vi "ReadXCANVersion.vi"() -> (1 "InstallTime":string, 2 "Version":string)   [LabVIEW 2015]
uses:
  <vilib>/registry/registry.llb/Registry RtKey.ctl
  <vilib>/registry/registry.llb/Registry SAM.ctl
  <vilib>/registry/registry.llb/Registry View.ctl
  <vilib>/registry/registry.llb/Read Registry Value Simple STR.vi
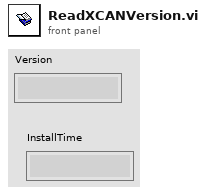
[diagram p1: front panel]
types:
  T1 = typedef "Registry View.ctl" = u16
  T2 = typedef "Registry SAM.ctl" = enum32{"KEY_QUERY_VALUE", "KEY_SET_VALUE", "KEY_CREATE_SUB_KEY", "KEY_ENUMERATE_SUB_KEYS", "KEY_NOTIFY", "KEY_CREATE_LINK", "KEY_READ", "KEY_WRITE", "KEY_ALL_ACCESS", "KEY_READ | KEY_WRITE"}
  T3 = typedef "Registry RtKey.ctl" = enum32{"HKEY_CLASSES_ROOT", "HKEY_CURRENT_USER", "HKEY_LOCAL_MACHINE", "HKEY_USERS", "HKEY_PERFORMANCE_DATA", "HKEY_CURRENT_CONFIG", "HKEY_DYN_DATA"}
  T4 = typedef "Registry refnum.ctl" = refnum<k1>
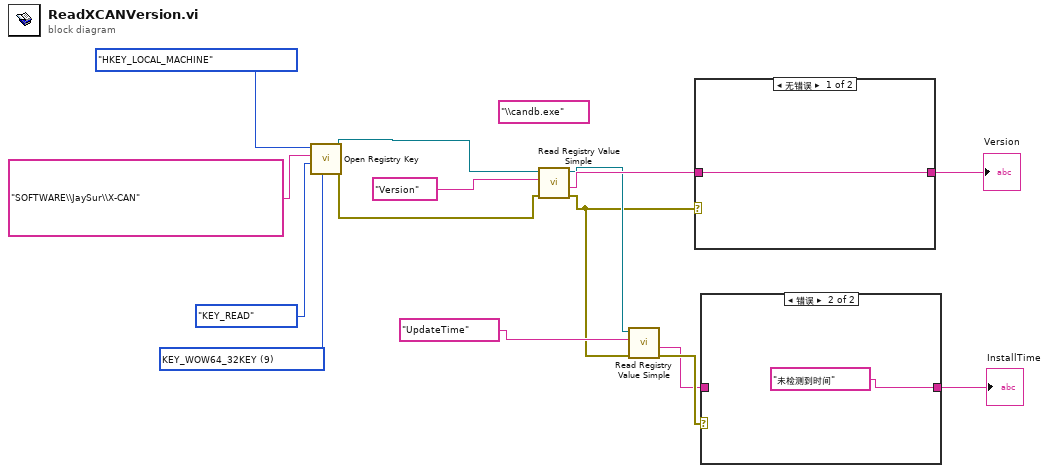
[diagram p0: block diagram]
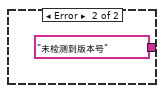
[diagram p3: hidden frame]
diagram:
  (unwired) "\\candb.exe" ("字符串")
  w12 = T1 9 items=["Default"=0, "KEY_WOW64_64KEY"=8, "KEY_WOW64_32KEY"=9] ("registry view")
  n1 = call <vilib>:"Open Registry Key.vi"("registry view"=w12, "security access mask (KEY_READ | KEY_WRITE)"=Registry_SAM."KEY_READ", "subkey"="SOFTWARE\\JaySur\\X-CAN", "root key (HKEY_LOCAL_MACHINE)"=Registry_RtKey."HKEY_LOCAL_MACHINE") -> ("error out"=w9:errorcluster, "refnum out"=w11:T4)  [unwired: 6 in]
  n2 = call-poly <vilib>:"Read Registry Value Simple.vi"("error in (no error)"=w9, "value"="Version", "refnum"=w11) -> ("error out"=w4:errorcluster, "String/Binary data"=w8:string, "refnum out"=w6:T4)  [unwired: 3 in, 1 out]
  n3 = call-poly <vilib>:"Read Registry Value Simple.vi"("error in (no error)"=w4, "value"="UpdateTime", "refnum"=w6) -> ("error out"=w3:errorcluster, "String/Binary data"=w2:string)  [unwired: 3 in, 2 out]
  n4 = case shown="无错误" w4 {
    tunnel: w8 -> [w16 _]
    tunnel: [w16 "未检测到版本号" ("String/Binary data")] -> w7
    frame No Error {
    }
    frame Error {
    }
  }
  "Version" <- w7
  n5 = case shown="错误" w3 {
    tunnel: w2 -> [w18 _]
    tunnel: [w18 "未检测到时间" ("String/Binary data")] -> w1
    frame No Error {
    }
    frame Error {
    }
  }
  "InstallTime" <- w1
